vi "Initialize From Config.vi"(0 "Engine Data":T1={"Loop Info"={"Processor"=-2, "Priority"=0}, "Main Tag Data"={"Double"=[], "Single"=[], "I64"=[], "I32"=[], "I16"=[], "I8"=[], "U64"=[], "U32"=[], "U16"=[], "U8"=[], "Boolean"=[], "String"=[], "Array of Double"=[], "Array of Single"=[], "Array of I64"=[], "Array of I32"=[], "Array of I16"=[], "Array of I8"=[], "Array of U64"=[], "Array of U32"=[], "Array of U16"=[], "Array of U8"=[], "Array of Boolean"=[], "Array of String"=[]}, "Module Info"={"Tag Bus Modules"=[], "Execute?"=[], "Input Method Indices"=[], "Process Method Indices"=[], "Output Method Indices"=[], "Input Transfer Specifications"=[], "Parameter Transfer Specifications"=[], "Result Transfer Specifications"=[], "Output Transfer Specifications"=[], "Module Errors"=[], "Module Decimation"=[], "Module Decimation Indices"=[], "Error Queue"=refnum, "Module Error Configuration"=[], "Module Errors (n-1)"=[]}, "engine timing source"=refnum, "timing policy"=enum."nonblocking", "async execution info"={"Tag Bus Modules"=[], "Execute?"=[], "Input Method Indices"=[], "Process Method Indices"=[], "Output Method Indices"=[], "Input Transfer Specifications"=[], "Parameter Transfer Specifications"=[], "Result Transfer Specifications"=[], "Output Transfer Specifications"=[], "Module Errors"=[], "Module Decimation"=[], "Module Decimation Indices"=[], "Error Queue"=refnum, "Module Error Configuration"=[], "comm errors"=[]}, "status reporting"={"late index (bool)"=-1, "late count (U32)"=-1, "current dt ns(U64)"=-1, "synchronous modules"=[], "asynchronous modules"=[]}, "Timing Source dt"=0}, 5 "Engine Configuration":refnum<class "Standard Engine Configuration.lvclass">, 7 "Modules":refnum<class "TBM module execution interface.lvclass">[](array[class]), 9 "Module Configurations":refnum<class "TBM module configuration.lvclass">[](array[class]), 11 "error in":errorcluster) -> (4 "Engine Data Out":T1={"Loop Info"={"Processor"=-2, "Priority"=0}, "Main Tag Data"={"Double"=[], "Single"=[], "I64"=[], "I32"=[], "I16"=[], "I8"=[], "U64"=[], "U32"=[], "U16"=[], "U8"=[], "Boolean"=[], "String"=[], "Array of Double"=[], "Array of Single"=[], "Array of I64"=[], "Array of I32"=[], "Array of I16"=[], "Array of I8"=[], "Array of U64"=[], "Array of U32"=[], "Array of U16"=[], "Array of U8"=[], "Array of Boolean"=[], "Array of String"=[]}, "Module Info"={"Tag Bus Modules"=[], "Execute?"=[], "Input Method Indices"=[], "Process Method Indices"=[], "Output Method Indices"=[], "Input Transfer Specifications"=[], "Parameter Transfer Specifications"=[], "Result Transfer Specifications"=[], "Output Transfer Specifications"=[], "Module Errors"=[], "Module Decimation"=[], "Module Decimation Indices"=[], "Error Queue"=refnum, "Module Error Configuration"=[], "Module Errors (n-1)"=[]}, "engine timing source"=refnum, "timing policy"=enum."nonblocking", "async execution info"={"Tag Bus Modules"=[], "Execute?"=[], "Input Method Indices"=[], "Process Method Indices"=[], "Output Method Indices"=[], "Input Transfer Specifications"=[], "Parameter Transfer Specifications"=[], "Result Transfer Specifications"=[], "Output Transfer Specifications"=[], "Module Errors"=[], "Module Decimation"=[], "Module Decimation Indices"=[], "Error Queue"=refnum, "Module Error Configuration"=[], "comm errors"=[]}, "status reporting"={"late index (bool)"=-1, "late count (U32)"=-1, "current dt ns(U64)"=-1, "synchronous modules"=[], "asynchronous modules"=[]}, "Timing Source dt"=0}, 15 "error out":errorcluster)   [LabVIEW 2013, in "Standard Engine Runtime.lvclass"]
doc: "This VI contains all of the logic necessary for configuring the engine based on a given engine configuration, and an array of modules with their configurations. \n\nFirst it allows the modules to finish configuring themselves by calling their dynamic configuration and mapping functions. \n\nThen it calls the Init method for each module and initializes their channel data space as well as the engine's tag data space. \n\nIt also initializes all of the other features of the engine including the timing source, decimation, error handling, execution order, etc."
uses:
  Standard Engine Runtime.lvclass
  Engine Data.ctl
  <vilib>/NI/Module Timing Source/timing source/TBM timing source.lvclass
  Configuration/Loop Info.ctl
  <vilib>/NI/Tag Bus/table/data table.ctl
  Module Execution Info.ctl
  <vilib>/NI/Tag Bus Module Framework/runtime/TBM module execution interface.lvclass
  Data Table with Transfer Spec.ctl
  <vilib>/NI/Tag Bus/table/transfer specification.ctl
  <vilib>/NI/Tag Bus/tag/Data Type.ctl
  Configuration/Module Decimation.ctl
  Configuration/Module Error Configuration.ctl
  Configuration/Error Actions By Category.ctl
  <vilib>/NI/Tag Bus Module Framework/runtime/error classification.ctl
  Configuration/Error Actions.ctl
  Configuration/timing policy.ctl
  async execution info.ctl
  asynchronous process data.ctl
  async command notification.ctl
  <vilib>/NI/Tag Bus Module Framework/runtime/execution settings.ctl
  async error info.ctl
  status reporting data.ctl
  module status reporting.ctl
  Configuration/Standard Engine Configuration.lvclass
  <vilib>/NI/Tag Bus Module Framework/module configuration/TBM module configuration.lvclass
  Configuration/Standard Engine Configuration.lvclass/Standard Engine Configuration.ctl
  <vilib>/NI/Configuration Framework/serializable configuration/NISE_CEF_serializable configuration.lvclass/NISE_CEF_serializable configuration.ctl
  <vilib>/NI/Configuration Framework/serializable configuration/NISE_CEF_serializable configuration.lvclass
  <vilib>/NI/Module Timing Source/standard timing source/ms timing source.lvclass
  <vilib>/NI/Module Timing Source/usec timing source/usec timing source.lvclass
  <vilib>/NI/Module Timing Source/scan engine timing source/scan engine timing source.lvclass
  <vilib>/NI/Module Execution Interface/Engine Configuration/engine configuration.lvclass/engine configuration.ctl
  <vilib>/NI/Tag Bus/dictionary/data dictionary.lvclass/data dictionary.ctl
  <vilib>/NI/Tag Bus/dictionary/lookup polymorphs/locate I32.vi
  Configuration/Read timing policy.vi
  Configuration/Read Timing Source Type.vi
  Configuration/Read Processor.vi
  Configuration/Read Master Timing Module.vi
  <vilib>/NI/Tag Bus/dictionary/search/find data index.vi
  <vilib>/NI/Tag Bus/dictionary/search/search string list.vi
  Configuration/Read Timing Source dt.vi
  Configuration/Find Module Specific Config.vi
  <vilib>/Utility/error.llb/Error Cluster From Error Code.vi
  <vilib>/NI/Tag Bus/dictionary/tag not found.vi
  <vilib>/Utility/RT CPU pool selections.ctl
  <vilib>/NI/Tag Bus/dictionary/data dictionary.lvclass
  <vilib>/NI/Module Execution Interface/Engine Configuration/engine configuration.lvclass
  <vilib>/NI/Module Execution Interface/Engine Runtime/Engine Runtime Interface.lvclass
  <vilib>/NI/Tag Bus/tag/tag descriptor.lvclass
  <vilib>/NI/Tag Bus/table/data table.lvlib
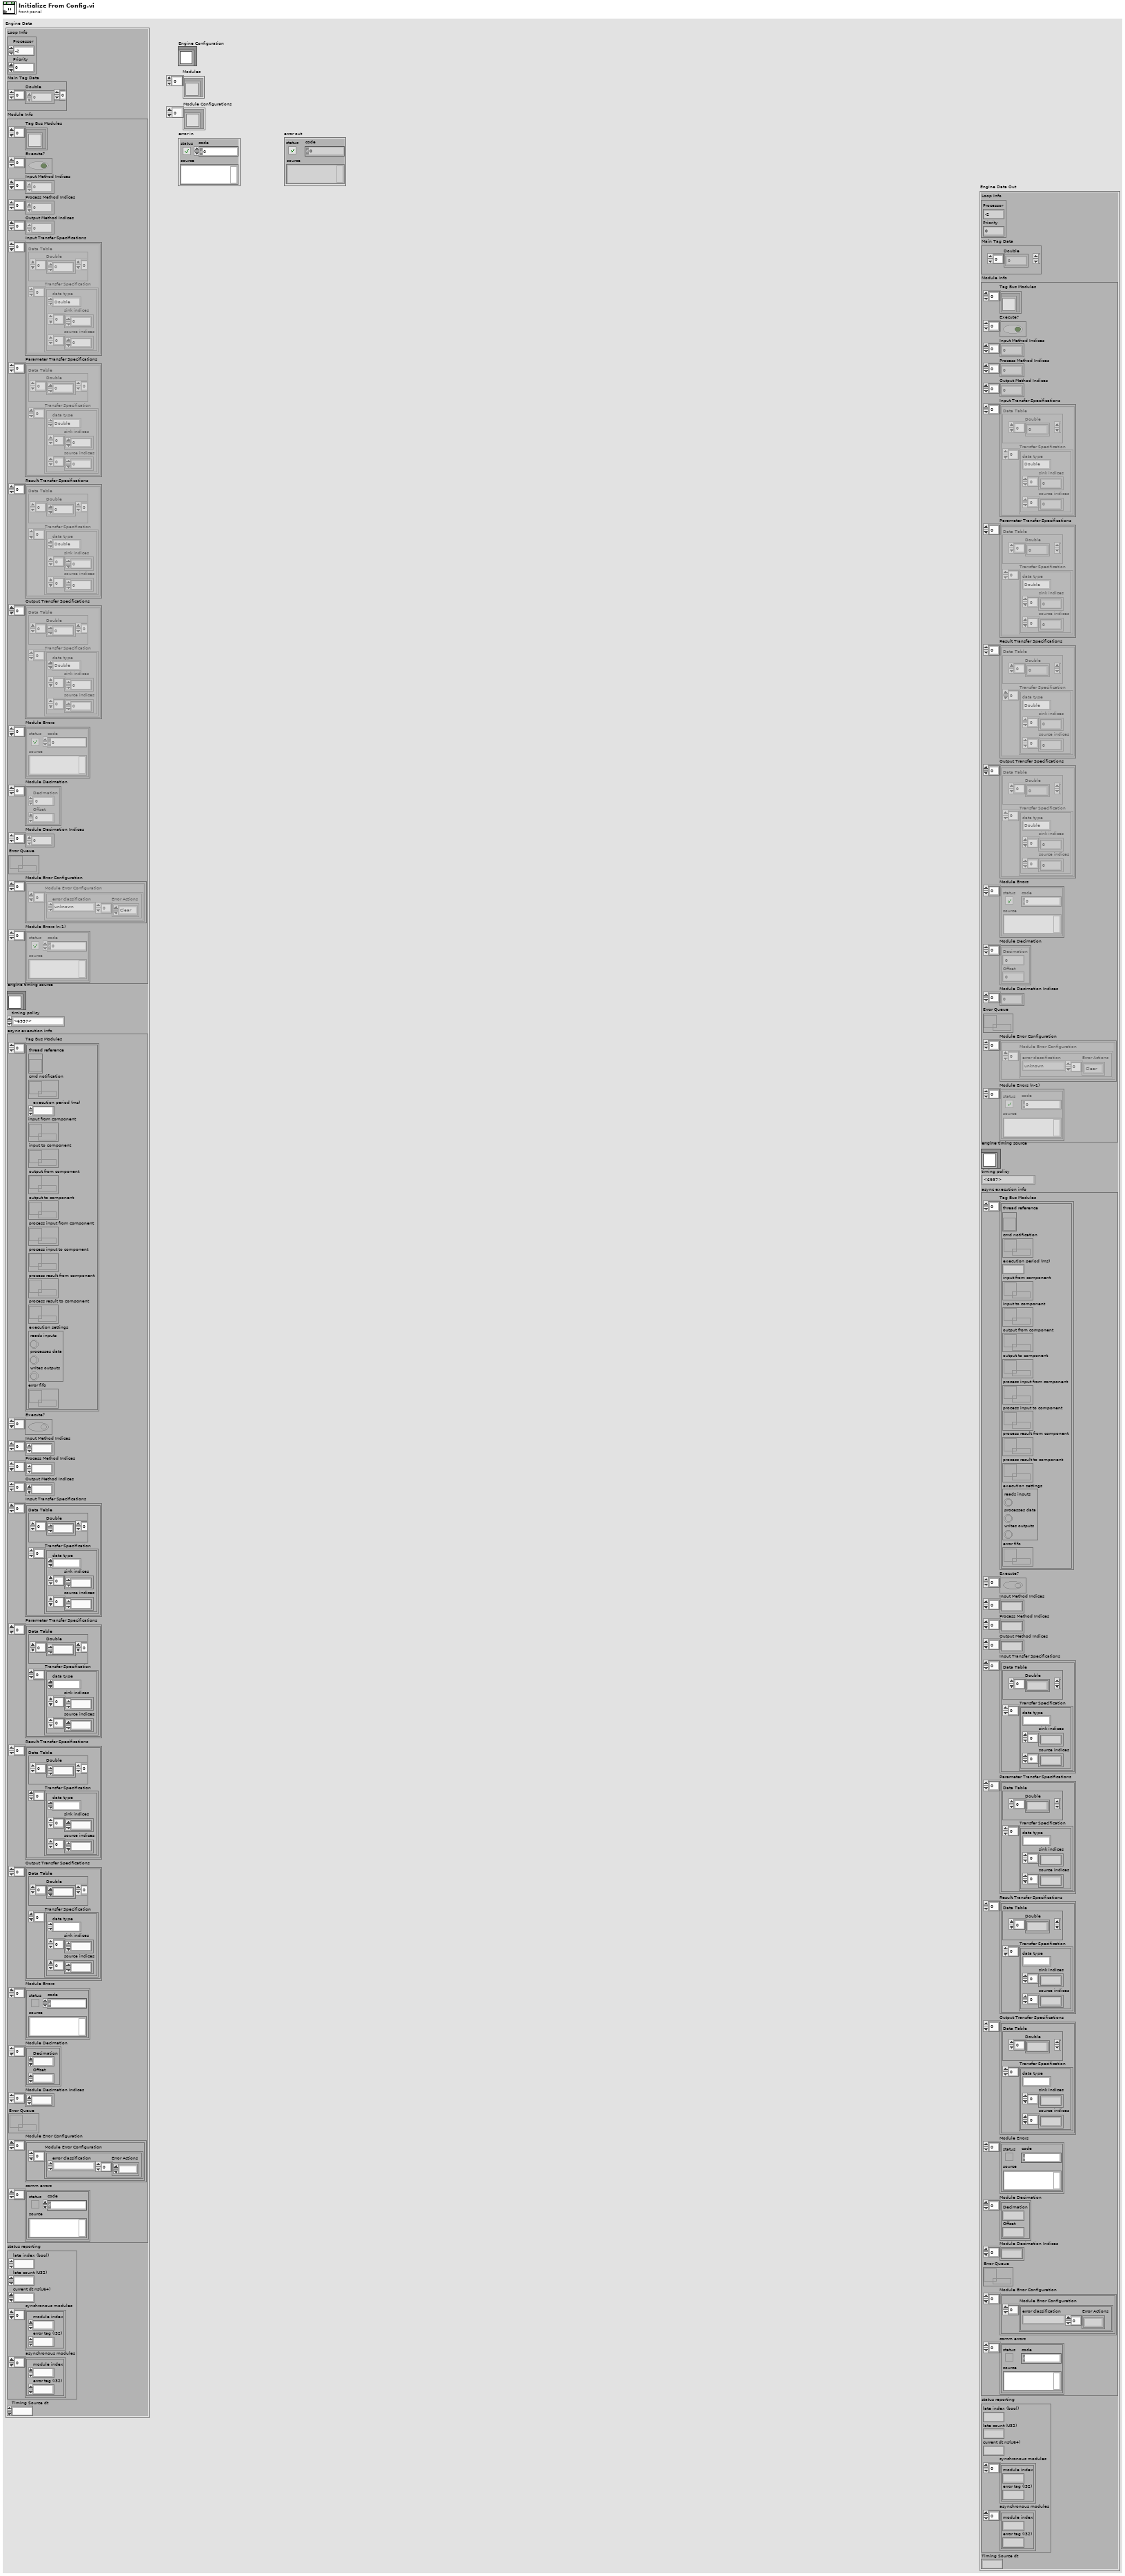
[diagram p1: front panel]
types:
  T1 = typedef "Standard Engine Runtime.lvclass/Engine Data.ctl" = cluster{"Loop Info":T2, "Main Tag Data":T3, "Module Info":T4, "engine timing source":refnum<class "TBM timing source.lvclass">, "timing policy":T13, "async execution info":T14, "status reporting":T17, "Timing Source dt":u32}
  T2 = typedef "Standard Engine Configuration.lvclass/Loop Info.ctl" = cluster{"Processor":i32, "Priority":i32}
  T3 = typedef "tag bus.lvlib/data table.lvlib/data table.ctl" = cluster{"Double":dbl[], "Single":sgl[], "I64":i64[], "I32":i32[], "I16":i16[], "I8":i8[], "U64":u64[], "U32":u32[], "U16":u16[], "U8":u8[], "Boolean":bool[], "String":string[], "Array of Double":cluster{"DBL Array":dbl[]}[], "Array of Single":cluster{"SGL Array":sgl[]}[], "Array of I64":cluster{"I64 Array":i64[]}[], "Array of I32":cluster{"I32 Array":i32[]}[], "Array of I16":cluster{"I16 Array":i16[]}[], "Array of I8":cluster{"I8 Array":i8[]}[], "Array of U64":cluster{"U64 Array":u64[]}[], "Array of U32":cluster{"U32 Array":u32[]}[], "Array of U16":cluster{"U16 Array":u16[]}[], "Array of U8":cluster{"U8 Array":u8[]}[], "Array of Boolean":cluster{"Boolean Array":bool[]}[], "Array of String":cluster{"String Array":string[]}[]}
  T4 = typedef "Standard Engine Runtime.lvclass/Module Execution Info.ctl" = cluster{"Tag Bus Modules":refnum<class "TBM module execution interface.lvclass">[], "Execute?":bool[], "Input Method Indices":i32[], "Process Method Indices":i32[], "Output Method Indices":i32[], "Input Transfer Specifications":T5[], "Parameter Transfer Specifications":T5[], "Result Transfer Specifications":T5[], "Output Transfer Specifications":T5[], "Module Errors":errorcluster[], "Module Decimation":T8[], "Module Decimation Indices":i32[], "Error Queue":refnum<queue>, "Module Error Configuration":T9[], "Module Errors (n-1)":errorcluster[]}
  T5 = typedef "Standard Engine Runtime.lvclass/Data Table with Transfer Spec.ctl" = cluster{"Data Table":T3, "Transfer Specification":T6[]}
  T6 = typedef "tag bus.lvlib/data table.lvlib/transfer specification.ctl" = cluster{"data type":T7, "sink indices":i32[], "source indices":i32[]}
  T7 = typedef "tag bus.lvlib/tag descriptor.lvclass/Data Type.ctl" = enum16{"Double", "Single", "I64", "I32", "I16", "I8", "U64", "U32", "U16", "U8", "Boolean", "String", "Array of Double", "Array of Single", "Array of I64", "Array of I32", "Array of I16", "Array of I8", "Array of U64", "Array of U32", "Array of U16", "Array of U8", "Array of Boolean", "Array of String"}
  T8 = typedef "Standard Engine Configuration.lvclass/Module Decimation.ctl" = cluster{"Decimation":u16, "Offset":u16}
  T9 = typedef "Standard Engine Configuration.lvclass/Module Error Configuration.ctl" = cluster{"Module Error Configuration":T10[]}
  T10 = typedef "Standard Engine Configuration.lvclass/Error Actions By Category.ctl" = cluster{"error classification":T11, "Error Actions":T12[]}
  T11 = typedef "TBM module execution interface.lvclass/error classification.ctl" = enum16{"unknown", "none", "trivial", "recoverable", "critical"}
  T12 = typedef "Standard Engine Configuration.lvclass/Error Actions.ctl" = enum16{"Clear", "Notify", "Stop Component", "Stop Engine", "Safe State", "Attempt Recovery"}
  T13 = typedef "Standard Engine Configuration.lvclass/timing policy.ctl" = enum16{"strict determinism", "nonblocking", "nondeterministic inline"}
  T14 = typedef "Standard Engine Runtime.lvclass/async execution info.ctl" = cluster{"Tag Bus Modules":T15[], "Execute?":bool[], "Input Method Indices":i32[], "Process Method Indices":i32[], "Output Method Indices":i32[], "Input Transfer Specifications":T5[], "Parameter Transfer Specifications":T5[], "Result Transfer Specifications":T5[], "Output Transfer Specifications":T5[], "Module Errors":errorcluster[], "Module Decimation":T8[], "Module Decimation Indices":i32[], "Error Queue":refnum<queue>, "Module Error Configuration":T9[], "comm errors":errorcluster[]}
  T15 = typedef "Standard Engine Runtime.lvclass/asynchronous process data.ctl" = cluster{"thread reference":refnum<vi>, "cmd notification":refnum<k33>, "execution period (ms)":i32, "input from component":refnum<queue>, "input to component":refnum<queue>, "output from component":refnum<queue>, "output to component":refnum<queue>, "process input from component":refnum<queue>, "process input to component":refnum<queue>, "process result from component":refnum<queue>, "process result to component":refnum<queue>, "execution settings":T16, "error fifo":refnum<k33>}
  T16 = typedef "TBM module execution interface.lvclass/execution settings.ctl" = cluster{"reads inputs":bool, "processes data":bool, "writes outputs":bool}
  T17 = typedef "Standard Engine Runtime.lvclass/status reporting data.ctl" = cluster{"late index (bool)":i32, "late count (U32)":i32, "current dt ns(U64)":i32, "synchronous modules":T18[], "asynchronous modules":T18[]}
  T18 = typedef "Standard Engine Runtime.lvclass/module status reporting.ctl" = cluster{"module index":i32, "error tag (I32)":i32}
  T19 = typedef "Standard Engine Configuration.lvclass/Supported Timing Sources.ctl" = enum16{"Use Module Timing Source", "1 kHz Clock", "1 MHz Clock", "Synchronize to Scan Engine"}
  T20 = cluster{"execution order priority":i32, "module index":i32}
  T21 = typedef "TBM channel.lvclass/data tables.ctl" = cluster{"input data":T22, "processing parameter":T22, "processing result":T22, "output data":T22}
  T22 = typedef "tag bus.lvlib/dictionary table pair.ctl" = cluster{"data dictionary":refnum<class "data dictionary.lvclass">, "data table":T3}
  T23 = typedef "Standard Engine Configuration.lvclass/timing reporting tags.ctl" = cluster{"late index (bool)":string, "late count index (U32)":string, "current dt ns(U64)":string}
  T24 = typedef "NI_Real-Time Target Support.lvlib/RT CPU pool selections.ctl" = enum16{"System & Timed Structures", "System", "Timed Structures", "Reserved"}
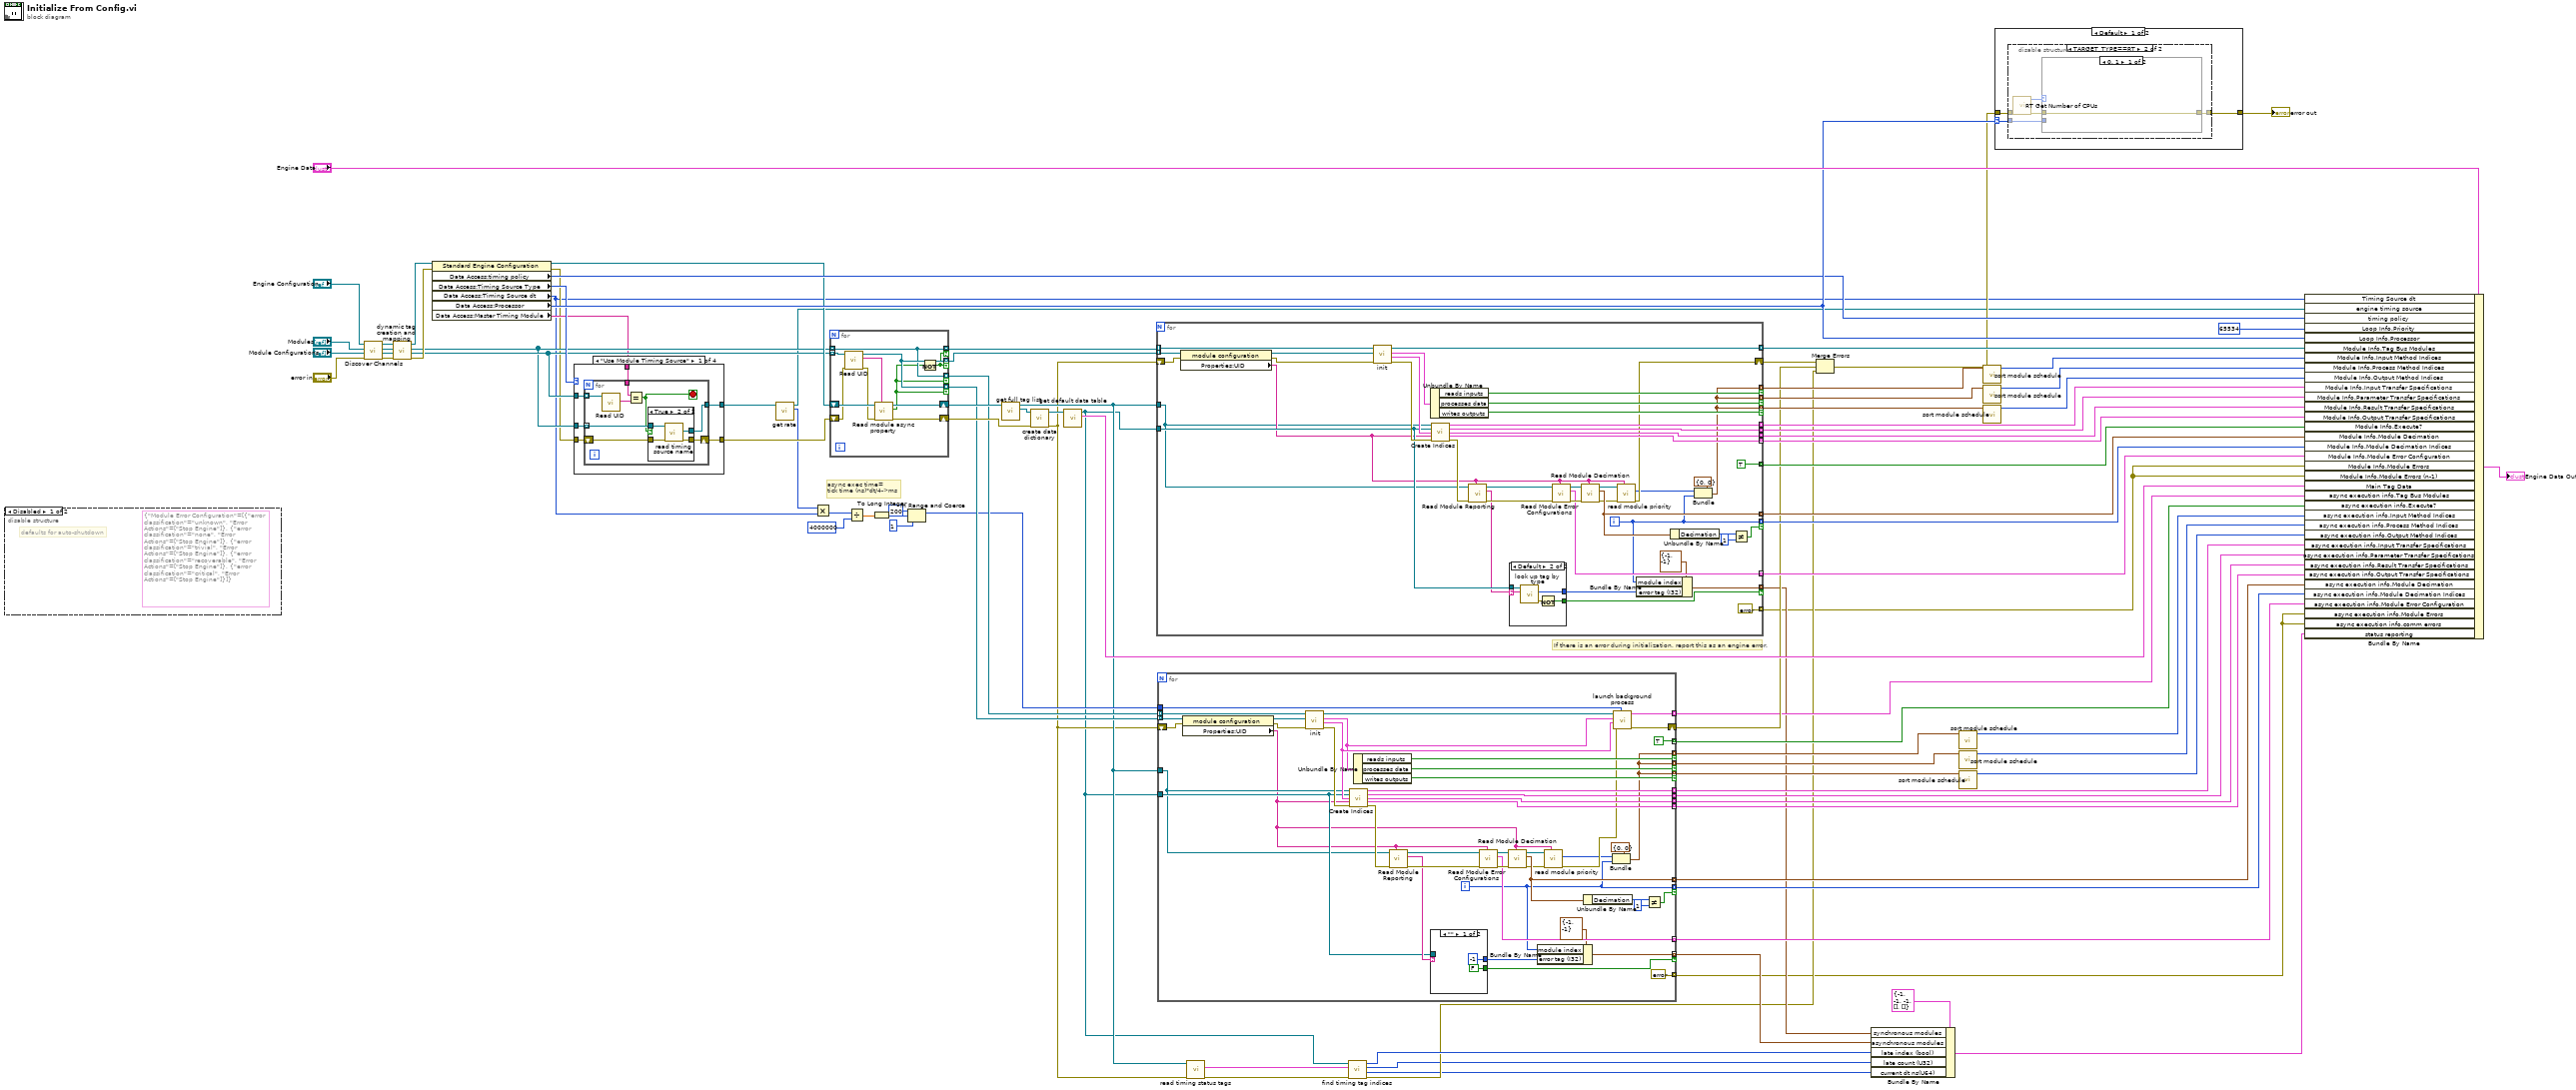
[diagram p0: block diagram]
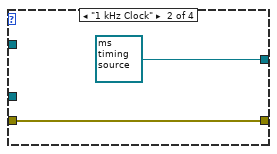
[diagram p3: hidden frame]
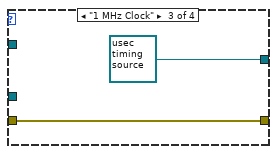
[diagram p4: hidden frame]
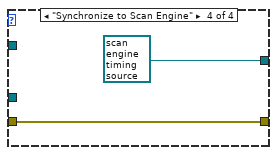
[diagram p5: hidden frame]
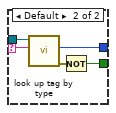
[diagram p6: hidden frame]
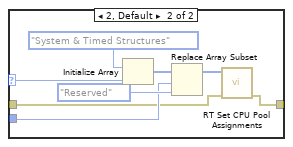
[diagram p9: hidden frame]
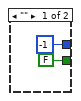
[diagram p11: hidden frame]
diagram:
  # "async exec time=\ntick time (ns)*dt/4->ms"
  # "If there is an error during initialization, report this as an engine error."
  n1 = disable-structure shown="Disabled" {
    frame Disabled {
      (unwired) T9 {"Module Error Configuration"=[{"error classification"=enum."unknown", "Error Actions"=[enum."Stop Engine"]}, {"error classification"=enum."none", "Error Actions"=[enum."Stop Engine"]}, {"error classification"=enum."trivial", "Error Actions"=[enum."Stop Engine"]}, {"error classification"=enum."recoverable", "Error Actions"=[enum."Stop Engine"]}, {"error classification"=enum."critical", "Error Actions"=[enum."Stop Engine"]}]} ("Module Error Configuration")
      # "defaults for auto-shutdown"
    }
    frame Enabled {
    }
  }
  n2 = call <vilib>:"Discover Channels.vi"("error in (no error)"="error in", "module configurations"="Module Configurations", "modules"="Modules", "engine configuration"="Engine Configuration") -> ("error out"=w75:errorcluster, "module configurations out"=w76:refnum<class "TBM module configuration.lvclass">[], "modules out"=w77:refnum<class "TBM module execution interface.lvclass">[], "engine configuration out"=w78:refnum<class "Standard Engine Configuration.lvclass">)  [unwired: 4 in]
  n3 = call <vilib>:"dynamic tag creation and mapping.vi"("error in"=w75, "module configurations"=w76, "modules"=w77, "engine configuration in"=w78) -> ("error out"=w69:errorcluster, "module configurations out"=w31:refnum<class "TBM module configuration.lvclass">[], "modules out"=w30:refnum<class "TBM module execution interface.lvclass">[], "engine configuration out"=w70:refnum<class "Standard Engine Configuration.lvclass">)  [unwired: 4 in]
  n4 = property class="Standard Engine Configuration"(reference=w70, error in=w69) -> (reference out=w56:refnum<class "Standard Engine Configuration.lvclass">, error out=w27:errorcluster, "Data Access:timing policy"=w57:T13, "Data Access:Timing Source Type"=w32:T19, "Data Access:Timing Source dt"=w1:u32, "Data Access:Processor"=w64:i32, "Data Access:Master Timing Module"=w29:string)
  n5 = case shown="\"Use Module Timing Source\"" w32 {
    tunnel: [w94 refnum<class "ms timing source.lvclass"> refnum ("ms timing source.lvclass") refnum<class "usec timing source.lvclass"> refnum ("usec timing source.lvclass") refnum<class "scan engine timing source.lvclass"> refnum ("scan engine timing source.lvclass")] -> w26
    tunnel: w31 -> [w97 _ _ _]
    tunnel: w30 -> [w96 _ _ _]
    tunnel: w29 -> [w95 _ _ _]
    tunnel: [w93 w111 w113 w115] -> w28
    tunnel: w27 -> [w92 w111 w113 w115]
    frame "Use Module Timing Source" {
      n6 = for {
        tunnel: w97 -> [w105] mode=indexing
        tunnel: w96 -> [w102] mode=indexing
        tunnel: w95 -> [w103]
        tunnel: [w100] -> w94
        shift-right: [w99] -> w93
        shift-left: w92 -> [w98]
        stop <- w101 stop-if-true
        n7 = call <vilib>:"Read UID.vi"("configuration in"=w105) -> ("instance id"=w104:string)  [unwired: 8 in, 2 out]
        n8 = Equal?(x=w103, y=w104) -> (x = y?=w101:bool)
        n9 = case shown="True" w101 {
          tunnel: w102 -> [_ w110]
          tunnel: [_ w109] -> w100
          tunnel: [w106 w108] -> w99
          tunnel: w98 -> [w106 w107]
          frame False {
          }
          frame True {
            n10 = call-dynamic "read timing source name.vi"("error in"=w107, "module in"=w110) -> ("error out"=w108:errorcluster, "timing source"=w109:refnum<class "TBM timing source.lvclass">)  [unwired: 7 in, 1 out]
          }
        }
      }
    }
    frame "1 kHz Clock" {
    }
    frame "1 MHz Clock" {
    }
    frame "Synchronize to Scan Engine" {
    }
  }
  n11 = call-dynamic "get rate.vi"("timing source in"=w26) -> ("period (ns)"=w24:i64, "timing source out"=w25:refnum<class "TBM timing source.lvclass">)  [unwired: 8 in, 1 out]
  n12 = Multiply(x=w24, y=w1) -> (x*y=w23:i64)
  n13 = for {
    tunnel: w31 -> [w127] mode=indexing
    tunnel: w30 -> [w122] mode=indexing
    shift-right: [w124] -> w55
    shift-left: w56 -> [w125]
    tunnel: [w123] -> w53 mode=indexing if=w118
    tunnel: [w122] -> w54 mode=indexing if=w118
    tunnel: [w123] -> w50 mode=indexing if=w117
    tunnel: [w122] -> w51 mode=indexing if=w117
    shift-right: [w121] -> w52
    shift-left: w28 -> [w119]
    n14 = call <vilib>:"Read UID.vi"("error in"=w119, "configuration in"=w127) -> ("error out"=w120:errorcluster, "instance id"=w126:string, "configuration out"=w123:refnum<class "TBM module configuration.lvclass">)  [unwired: 7 in]
    n15 = call "Read module async property.vi"("Module ID"=w126, "error in"=w120, "Standard Engine Repo Data in"=w125) -> ("error out"=w121:errorcluster, "async?"=w117:bool, "Standard Engine Repo Data out"=w124:refnum<class "Standard Engine Configuration.lvclass">)  [unwired: 6 in]
    n16 = Not(x=w117) -> (.not. x?=w118:bool)
  }
  n17 = Divide(x=w23, y=i64 4000000) -> (x/y=w21:dbl)
  n18 = To Long Integer(number=w21) -> (32bit integer=w20:i32)
  n19 = In Range and Coerce(upper limit=200, x=w20, lower limit=1) -> (coerced(x)=w19:i32)  [unwired: 1 out]
  n20 = call <vilib>:"get full tag list.vi"("engine configuration in"=w55) -> ("tag list"=w68:refnum<class "tag descriptor.lvclass">[], "engine configuration out"=w12:refnum<class "Standard Engine Configuration.lvclass">)  [unwired: 9 in]
  n21 = call <vilib>:"create data dictionary.vi"("error in"=w52, "system tags"=w68) -> ("error out"=w11:errorcluster, "data dictionary"=w67:refnum<class "data dictionary.lvclass">)  [unwired: 8 in]
  n22 = call <vilib>:"get default data table.vi"("data dictionary in"=w67) -> ("default data table"=w79:T3, "data dictionary out"=w8:refnum<class "data dictionary.lvclass">)  [unwired: 9 in]
  n23 = for {
    tunnel: w53 -> [w155] mode=indexing
    shift-right: [w145] -> w83
    shift-left: w11 -> [w151]
    tunnel: w54 -> [w170] mode=indexing
    tunnel: [w150] -> w91 mode=indexing
    tunnel: [w142] -> w58 mode=indexing if=w169
    tunnel: [w142] -> w61 mode=indexing if=w168
    tunnel: [w142] -> w63 mode=indexing if=w167
    tunnel: [w166] -> w89 mode=indexing
    tunnel: [w165] -> w88 mode=indexing
    tunnel: [w164] -> w87 mode=indexing
    tunnel: [w163] -> w86 mode=indexing
    tunnel: [TRUE] -> w85 mode=indexing
    tunnel: [w134] -> w84 mode=indexing if=w159
    tunnel: [w147] -> w80 mode=indexing
    tunnel: [w154] -> w81 mode=indexing
    tunnel: [errorcluster {"status"=FALSE, "code"=0, "source"=""} ("error constant")] -> w3 mode=indexing
    tunnel: w8 -> [w133]
    tunnel: w12 -> [w128]
    tunnel: [w135] -> w15 mode=indexing if=w131
    i -> [w134]
    n24 = property class="module configuration"(reference=w155, error in=w151) -> (reference out=w152:refnum<class "TBM module configuration.lvclass">, error out=w140:errorcluster, "Properties:UID"=w129:string)
    n25 = call-dynamic "init.vi"("error in"=w140, "module configuration"=w152, "module in"=w170) -> ("error out"=w162:errorcluster, "data allocations"=w156:T21, "execution settings"=w157:T16, "module out"=w150:refnum<class "TBM module execution interface.lvclass">)  [unwired: 5 in]
    n26 = Unbundle By Name(w157) -> ("reads inputs"=w169:bool, "processes data"=w168:bool, "writes outputs"=w167:bool)
    n27 = call "Create Indices.vi"("Standard Engine Configuration"=w128, "main data dictionary"=w133, "data description"=w156, "Module ID"=w129, "error in"=w162) -> ("Input Transfer Specification"=w166:T5, "Parameter Transfer Specifcation"=w165:T5, "Result Transfer Specifcation"=w164:T5, "Output Transfer Specifcation"=w163:T5, "error out"=w139:errorcluster)  [unwired: 6 in]
    n28 = call "Read Module Reporting.vi"("Module ID"=w129, "error in"=w139, "Standard Engine Repo Data in"=w128) -> ("error out"=w138:errorcluster, "error tag"=w130:string, "Standard Engine Repo Data out"=w137:refnum<class "Standard Engine Configuration.lvclass">)  [unwired: 6 in]
    n29 = case shown="Default" w130 {
      selector: w130 -> [_ w173]
      tunnel: w133 -> [_ w177]
      tunnel: [-1 ("index") w176] -> w132
      tunnel: [FALSE w174] -> w131
      frame "" {
      }
      frame Default {
        n30 = call-poly <vilib>:"look up tag by type.vi"("name"=w173, "data dictionary in"=w177) -> ("error out"=w175:errorcluster, "index"=w176:i32)  [unwired: 7 in, 1 out]
        n31 = Not(x=w175) -> (.not. x?=w174:bool)
      }
    }
    n32 = call "Read Module Error Configurations.vi"("Module ID"=w129, "error in"=w138, "Standard Engine Repo Data in"=w137) -> ("error out"=w148:errorcluster, "Module Error Configuration"=w147:T9, "Standard Engine Repo Data out"=w149:refnum<class "Standard Engine Configuration.lvclass">)  [unwired: 6 in]
    n33 = call "Read Module Decimation.vi"("Module ID"=w129, "error in"=w148, "Standard Engine Repo Data in"=w149) -> ("error out"=w146:errorcluster, "Module Decimation"=w154:T8, "Standard Engine Repo Data out"=w144:refnum<class "Standard Engine Configuration.lvclass">)  [unwired: 6 in]
    n34 = call "read module priority.vi"("Module ID"=w129, "error in"=w146, "Standard Engine Repo Data in"=w144) -> ("error out"=w145:errorcluster, "execution order priority"=w143:i32)  [unwired: 6 in, 1 out]
    n35 = Bundle By Name(cluster=T18 {"module index"=-1, "error tag (I32)"=-1} ("module status report"), "module index"=w134, "error tag (I32)"=w132) -> (w135:T18)
    n36 = Unbundle By Name(w154) -> ("Decimation"=w153:u16)
    n37 = Bundle(cluster=T20 {"execution order priority"=0, "module index"=0} ("priority cluster"), "execution order priority"=w143, "module index"=w134) -> (w142:T20)
    n38 = Not Equal?(x=w153, y=u16 1) -> (x != y?=w159:bool)
  }
  n39 = for {
    tunnel: w50 -> [w210] mode=indexing
    shift-right: [w195] -> w47
    shift-left: w11 -> [w206]
    tunnel: w51 -> [w223] mode=indexing
    tunnel: [w198] -> w44 mode=indexing if=w222
    tunnel: [w198] -> w45 mode=indexing if=w221
    tunnel: [w198] -> w46 mode=indexing if=w220
    tunnel: [w219] -> w39 mode=indexing
    tunnel: [w218] -> w38 mode=indexing
    tunnel: [w217] -> w37 mode=indexing
    tunnel: [w216] -> w36 mode=indexing
    tunnel: [TRUE] -> w42 mode=indexing
    tunnel: [w181] -> w34 mode=indexing if=w212
    tunnel: [w203] -> w49 mode=indexing
    tunnel: [w209] -> w35 mode=indexing
    tunnel: [errorcluster {"status"=FALSE, "code"=0, "source"=""} ("error constant")] -> w2 mode=indexing
    tunnel: w8 -> [w182]
    tunnel: w12 -> [w180]
    tunnel: [w194] -> w33 mode=indexing
    tunnel: w19 -> [w191]
    tunnel: [w186] -> w14 mode=indexing if=w184
    i -> [w181]
    n40 = property class="module configuration"(reference=w210, error in=w206) -> (reference out=w207:refnum<class "TBM module configuration.lvclass">, error out=w196:errorcluster, "Properties:UID"=w179:string)
    n41 = call-dynamic "init.vi"("error in"=w196, "module configuration"=w207, "module in"=w223) -> ("error out"=w215:errorcluster, "data allocations"=w193:T21, "execution settings"=w192:T16, "module out"=w178:refnum<class "TBM module execution interface.lvclass">)  [unwired: 5 in]
    n42 = call "Create Indices.vi"("Standard Engine Configuration"=w180, "main data dictionary"=w182, "data description"=w193, "Module ID"=w179, "error in"=w215) -> ("Input Transfer Specification"=w219:T5, "Parameter Transfer Specifcation"=w218:T5, "Result Transfer Specifcation"=w217:T5, "Output Transfer Specifcation"=w216:T5, "error out"=w190:errorcluster)  [unwired: 6 in]
    n43 = Unbundle By Name(w192) -> ("reads inputs"=w222:bool, "processes data"=w221:bool, "writes outputs"=w220:bool)
    n44 = call "Read Module Reporting.vi"("Module ID"=w179, "error in"=w190, "Standard Engine Repo Data in"=w180) -> ("error out"=w189:errorcluster, "error tag"=w183:string, "Standard Engine Repo Data out"=w188:refnum<class "Standard Engine Configuration.lvclass">)  [unwired: 6 in]
    n45 = case shown="\"\"" w183 {
      selector: w183 -> [_ w226]
      tunnel: w182 -> [_ w230]
      tunnel: [-1 ("index") w229] -> w185
      tunnel: [FALSE w227] -> w184
      frame "" {
      }
      frame Default {
        n46 = call-poly <vilib>:"look up tag by type.vi"("name"=w226, "data dictionary in"=w230) -> ("error out"=w228:errorcluster, "index"=w229:i32)  [unwired: 7 in, 1 out]
        n47 = Not(x=w228) -> (.not. x?=w227:bool)
      }
    }
    n48 = call "Read Module Error Configurations.vi"("Module ID"=w179, "error in"=w189, "Standard Engine Repo Data in"=w188) -> ("error out"=w204:errorcluster, "Module Error Configuration"=w203:T9, "Standard Engine Repo Data out"=w205:refnum<class "Standard Engine Configuration.lvclass">)  [unwired: 6 in]
    n49 = call "Read Module Decimation.vi"("Module ID"=w179, "error in"=w204, "Standard Engine Repo Data in"=w205) -> ("error out"=w202:errorcluster, "Module Decimation"=w209:T8, "Standard Engine Repo Data out"=w200:refnum<class "Standard Engine Configuration.lvclass">)  [unwired: 6 in]
    n50 = Bundle By Name(cluster=T18 {"module index"=-1, "error tag (I32)"=-1} ("module status report"), "module index"=w181, "error tag (I32)"=w185) -> (w186:T18)
    n51 = call "read module priority.vi"("Module ID"=w179, "error in"=w202, "Standard Engine Repo Data in"=w200) -> ("error out"=w201:errorcluster, "execution order priority"=w199:i32)  [unwired: 6 in, 1 out]
    n52 = Unbundle By Name(w209) -> ("Decimation"=w208:u16)
    n53 = Bundle(cluster=T20 {"execution order priority"=0, "module index"=0} ("priority cluster"), "execution order priority"=w199, "module index"=w181) -> (w198:T20)
    n54 = call "launch background process.vi"("execution period (ms)"=w191, "error in"=w201, "data allocations"=w193, "execution settings"=w192, "module runtime"=w178) -> ("error out"=w195:errorcluster, "async data"=w194:T15)  [unwired: 5 in]
    n55 = Not Equal?(x=w208, y=u16 1) -> (x != y?=w212:bool)
  }
  n56 = call "read timing status tags.vi"("error in"=w11, "Standard Engine Configuration in"=w12) -> ("error out"=w9:errorcluster, "timing reporting"=w10:T23)  [unwired: 7 in, 1 out]
  n57 = call "find timing tag indices.vi"("error in"=w9, "timing reporting"=w10, "data dictionary in"=w8) -> ("error out"=w6:errorcluster, "dt ns"=w5:i32, "late count"=w4:i32, "late boolean"=w7:i32)  [unwired: 5 in]
  n58 = Merge Errors(w83, w47, w6) -> (w48:errorcluster)
  n59 = Bundle By Name(cluster=T17 {"late index (bool)"=-1, "late count (U32)"=-1, "current dt ns(U64)"=-1, "synchronous modules"=[], "asynchronous modules"=[]} ("status reporting"), "synchronous modules"=w15, "asynchronous modules"=w14, "late index (bool)"=w7, "late count (U32)"=w4, "current dt ns(U64)"=w5) -> (w13:T17)
  n60 = call "sort module schedule.vi"("priority array"=w44) -> ("sorted module indices"=w43:i32[])  [unwired: 10 in]
  n61 = call "sort module schedule.vi"("priority array"=w45) -> ("sorted module indices"=w40:i32[])  [unwired: 10 in]
  n62 = call "sort module schedule.vi"("priority array"=w46) -> ("sorted module indices"=w41:i32[])  [unwired: 10 in]
  n63 = call "sort module schedule.vi"("priority array"=w58) -> ("sorted module indices"=w59:i32[])  [unwired: 10 in]
  n64 = call "sort module schedule.vi"("priority array"=w61) -> ("sorted module indices"=w60:i32[])  [unwired: 10 in]
  n65 = call "sort module schedule.vi"("priority array"=w63) -> ("sorted module indices"=w62:i32[])  [unwired: 10 in]
  n66 = case shown="Default" w64 {
    selector: w64 -> [w231 _]
    tunnel: w48 -> [w233 w249]
    tunnel: [w232 w249] -> w82
    frame Default {
      n67 = disable-structure shown="TARGET_TYPE==RT" {
        disable-tunnel: w233 -> [w234 w238]
        disable-tunnel: w231 -> [_ w236]
        disable-tunnel: [w234 w235] -> w232
        frame condition #0 (active) {
        }
        frame condition #1 {
          n68 = call <vilib>:"RT Get Number of CPUs.vi"("error in (no error)"=w238) -> ("error out"=w237:errorcluster, "# of CPUs"=w239:u32)  [unwired: 9 in]
          n69 = case shown="0, 1" w239 {
            selector: w239 -> [_ w247]
            tunnel: w237 -> [w240 w242]
            tunnel: w236 -> [_ w244]
            tunnel: [w240 w241] -> w235
            frame 0, 1 {
            }
            frame 2, Default {
              n70 = Initialize Array(RT_CPU_pool_selections."System & Timed Structures" ("Enum"), w247) -> (w246:T24[])
              n71 = Replace Array Subset(array=w246, new element=RT_CPU_pool_selections."Reserved" ("new element/subarray"), index=w244) -> (w243:T24[])
              n72 = call <vilib>:"RT Set CPU Pool Assignments.vi"("error in (no error)"=w242, "CPU pools"=w243) -> ("error out"=w241:errorcluster)  [unwired: 6 in, 3 out]
            }
          }
        }
      }
    }
    frame -2 {
    }
  }
  "error out" <- w82
  n73 = Bundle By Name(cluster="Engine Data", "Timing Source dt"=w1, "engine timing source"=w25, "timing policy"=w57, "Loop Info.Priority"=65534, "Loop Info.Processor"=w64, "Module Info.Tag Bus Modules"=w91, "Module Info.Input Method Indices"=w59, "Module Info.Process Method Indices"=w60, "Module Info.Output Method Indices"=w62, "Module Info.Input Transfer Specifications"=w89, "Module Info.Parameter Transfer Specifications"=w88, "Module Info.Result Transfer Specifications"=w87, "Module Info.Output Transfer Specifications"=w86, "Module Info.Execute?"=w85, "Module Info.Module Decimation"=w81, "Module Info.Module Decimation Indices"=w84, "Module Info.Module Error Configuration"=w80, "Module Info.Module Errors"=w3, "Module Info.Module Errors (n-1)"=w3, "Main Tag Data"=w79, "async execution info.Tag Bus Modules"=w33, "async execution info.Execute?"=w42, "async execution info.Input Method Indices"=w43, "async execution info.Process Method Indices"=w40, "async execution info.Output Method Indices"=w41, "async execution info.Input Transfer Specifications"=w39, "async execution info.Parameter Transfer Specifications"=w38, "async execution info.Result Transfer Specifications"=w37, "async execution info.Output Transfer Specifications"=w36, "async execution info.Module Decimation"=w35, "async execution info.Module Decimation Indices"=w34, "async execution info.Module Error Configuration"=w49, "async execution info.Module Errors"=w2, "async execution info.comm errors"=w2, "status reporting"=w13) -> (→"Engine Data Out":T1)
